vi "FireBaseProyectoControlDePosicionPID_v2.vi"() -> ()   [LabVIEW 2025]
uses:
  <vilib>/httpClient/PUTBuffer.vi
  <vilib>/httpClient/LabVIEWHTTPClient.lvlib
panel:
  in  "Tab Control":T1(tab)
  out "OutputPWM":dbl
  out "PosicionActual":dbl
  out "ContadorInterrupcion":dbl
  in  "SetPoint  en grados Ctrl":dbl
  in  "Kp Ctrl":dbl=0.8899999999999997 format="%03.3f"
  in  "Ki Ctrl":dbl=0.7560000000000003 format="%01.3f"
  in  "Kd Ctrl":dbl=0.43500000000000116 format="%01.3f"
  out "ERROR Grafica":cluster{dbl, "PosicionActual":dbl}(graph)
  out "Body Desde el Servidor":string
  out "Header desde el servidor":string
  out "body hacia el servidor":string
  out "headers Hacia el Servidor":string
  out "Json Desde el Servidor":string
  out "Json al Servidor":string
  out "Comunicacion con el Servidor de FireBase":bool
  out "Comunicacion Con el server":string
  out "error out":errorcluster
  out "error out 2":errorcluster
  in  "stop":bool
  # "INTRUMENTACIoN VIRTUAL APLICADA"
  # "Control PID de un motor DC con conexión a FireBase"
  # "CONTROLES PID posicion de la flecha"
  # "Blanco es el error\nRojo la posicion Actual"
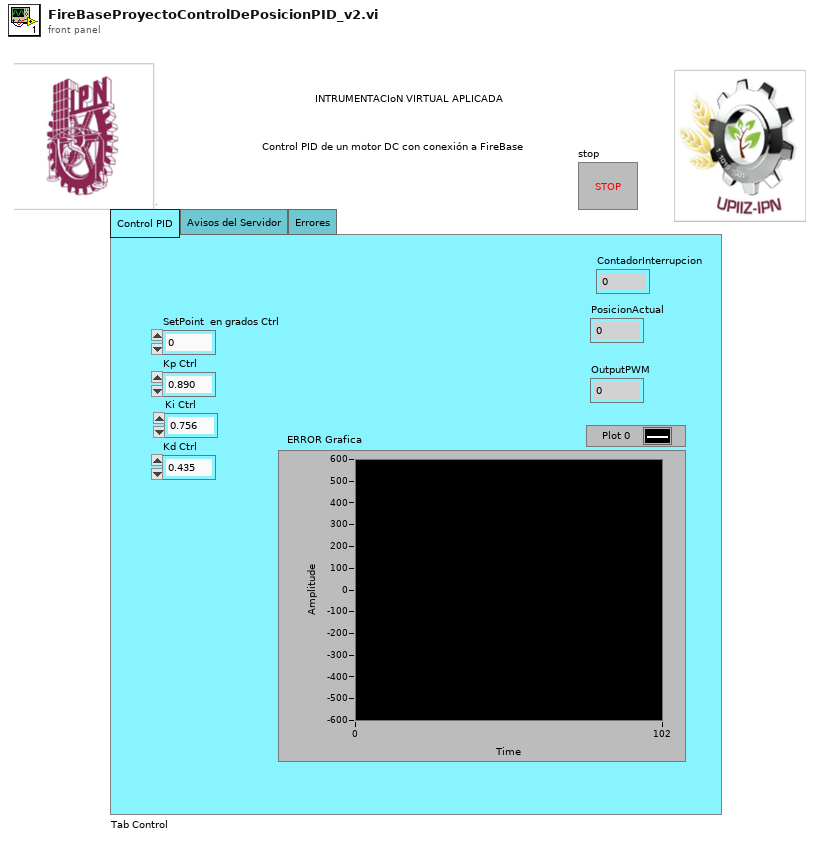
[diagram p1: front panel]
types:
  T1 = enum32{"Control PID", "Avisos del Servidor", "Errores"}
  T2 = cluster{"SetPoint":dbl, "Kp":dbl, "Ki":dbl, "Kd":dbl}
  T3 = cluster{"OutputPWM":dbl, "PosicionActual":dbl, "ContadorInterrupcion":dbl}
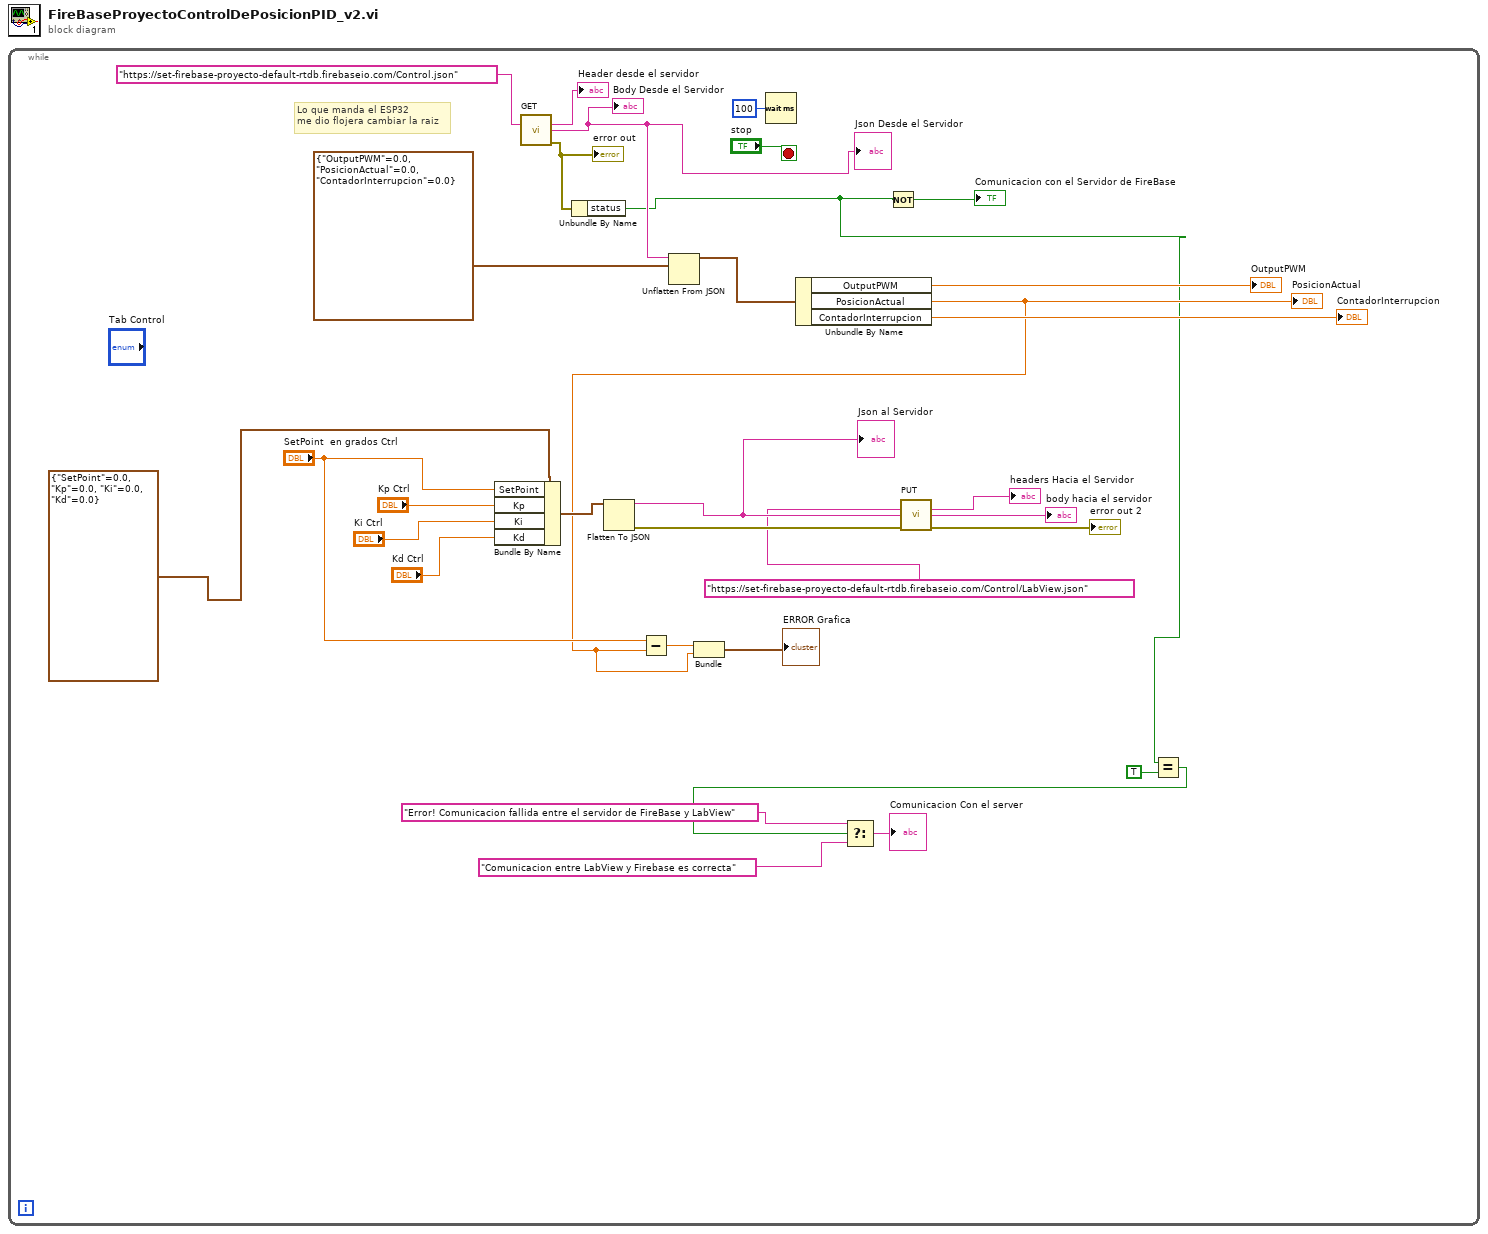
[diagram p0: block diagram]
diagram:
  n1 = while {
    stop <- "stop" stop-if-true
    # "Lo que manda el ESP32 \nme dio flojera cambiar la raiz"
    n2 = Bundle By Name "Bundle By Name"(cluster=T2 {"SetPoint"=0.0, "Kp"=0.0, "Ki"=0.0, "Kd"=0.0}, "SetPoint"="SetPoint  en grados Ctrl", "Kp"="Kp Ctrl", "Ki"="Ki Ctrl", "Kd"="Kd Ctrl") -> (w22:T2)
    n3 = call <vilib>:"GET.vi"("url"="https://set-firebase-proyecto-default-rtdb.firebaseio.com/Control.json") -> ("headers"=→"Header desde el servidor":string, "body"=w17:string, "error out"=w8:errorcluster)  [unwired: 11 in, 1 out]
    "error out" <- w8
    "Body Desde el Servidor" <- w17
    "Json Desde el Servidor" <- w17
    n4 = Unbundle By Name(w8) -> ("status"=w5:bool)
    n5 = Flatten To JSON(anything=w22) -> (JSON string=w18:string, 11:w23:errorcluster)  [unwired: 2 in]
    "Json al Servidor" <- w18
    n6 = Unflatten From JSON(JSON string=w17, type and defaults=T3 {"OutputPWM"=0.0, "PosicionActual"=0.0, "ContadorInterrupcion"=0.0}) -> (value=w29:T3)  [unwired: 5 in, 1 out]
    n7 = Wait (ms)(milliseconds to wait=u32 100) -> ()  [unwired: 1 out]
    n8 = Unbundle By Name "Unbundle By Name"(w29) -> ("OutputPWM"=→"OutputPWM":dbl, "PosicionActual"=w10:dbl, "ContadorInterrupcion"=→"ContadorInterrupcion":dbl)
    "PosicionActual" <- w10
    n9 = Subtract(x="SetPoint  en grados Ctrl", y=w10) -> (x-y=w11:dbl)
    n10 = Bundle(w11, "PosicionActual"=w10) -> (→"ERROR Grafica":cluster{dbl, "PosicionActual":dbl})  [unwired: 1 in]
    n11 = Not(x=w5) -> (.not. x?=→"Comunicacion con el Servidor de FireBase":bool)
    n12 = call-poly <vilib>:"PUT.vi"("url"="https://set-firebase-proyecto-default-rtdb.firebaseio.com/Control/LabView.json", "buffer"=w18, "error in (no error)"=w23) -> ("headers"=→"headers Hacia el Servidor":string, "body"=→"body hacia el servidor":string, "error out"=→"error out 2":errorcluster)  [unwired: 9 in, 1 out]
    n13 = Equal?(x=w5, y=TRUE) -> (x = y?=w6:bool)
    n14 = Select(t="Error! Comunicacion fallida entre el servidor de FireBase y LabView", s=w6, f="Comunicacion entre LabView y Firebase es correcta") -> (s? t:f=→"Comunicacion Con el server":string)
  }
